vi "Get All VI Data.vi"(8 "error in (no error)":errorcluster, 11 "Path":path) -> (0 "error out":errorcluster, 2 "Displayed Indices":i32[](array[numeric]), 3 "VI Data":T1[](array[typedef]))   [LabVIEW 2023, in "VI Properties Editor.lvlib"]
doc: "Gets all VI data from the source of VIs located at <B>Path</B>."
uses:
  VI Properties Editor.lvlib
  CTLs/VI Data.ctl
  CTLs/VI Properties.ctl
  <vilib>/picture/picture.llb/imagedata.ctl
  CTLs/Control Properties.ctl
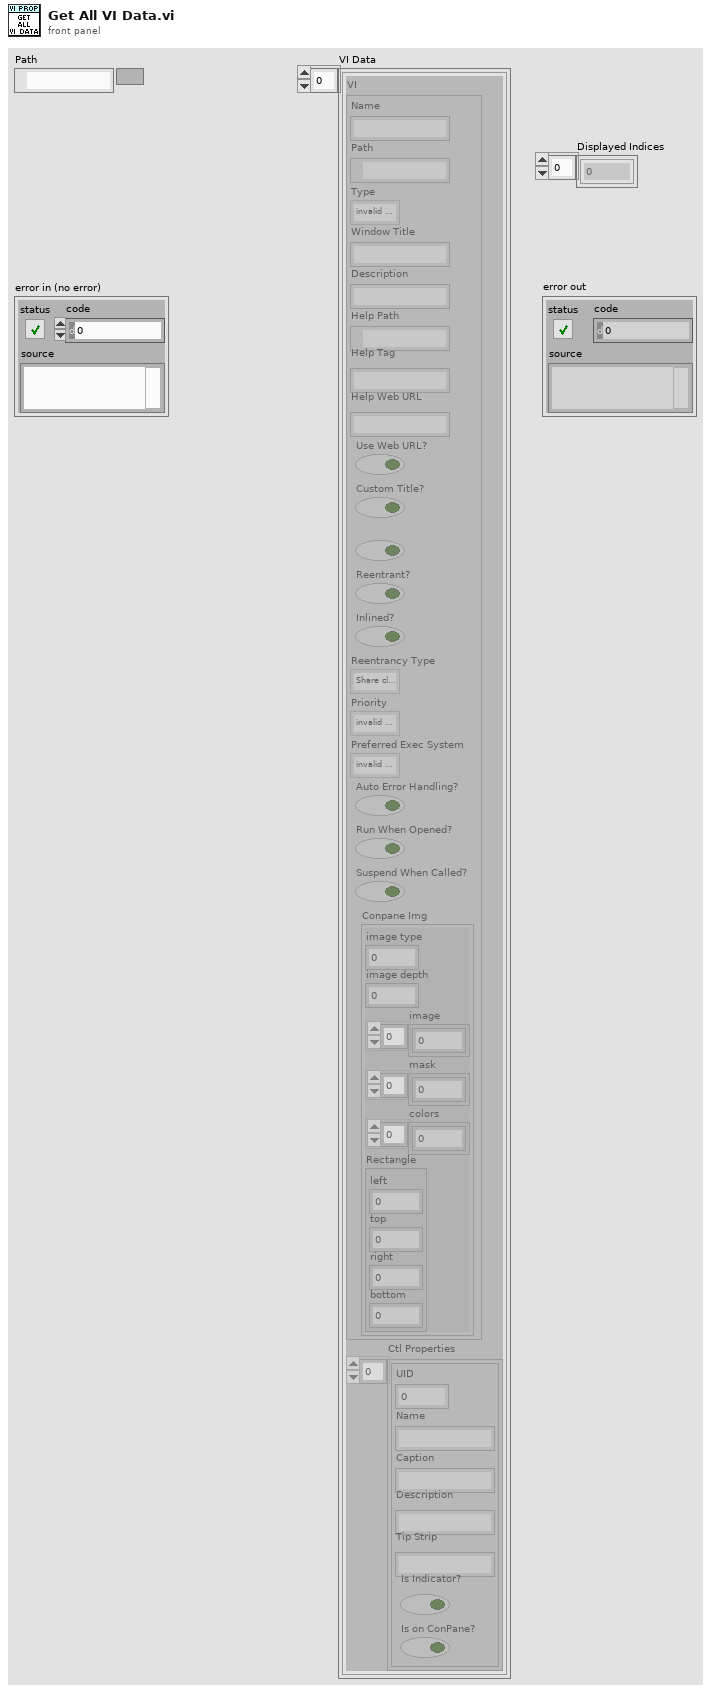
[diagram p1: front panel]
types:
  T1 = typedef "VI Properties Editor.lvlib/VI Data.ctl" = cluster{"VI":T2, "Ctl Properties":T4[]}
  T2 = typedef "VI Properties Editor.lvlib/VI Properties.ctl" = cluster{"Name":string, "Path":path, "Type":enum32{"invalid VI type", "Standard VI", "Control VI", "Global VI", "Polymorphic VI", "Configuration VI", "SubSystem", "Facade VI", "Method VI", "Statechart Diagram VI"}, "Window Title":string, "Description":string, "Help Path":path, "Help Tag":string, "Help Web URL":string, "Use Web URL?":bool, "Custom Title?":bool, "Allow Debugging?":bool, "Reentrant?":bool, "Inlined?":bool, "Reentrancy Type":enum16{"Share clones between instances", "Preallocate clone for each instance"}, "Priority":enum32{"invalid priority", "background priority", "normal priority", "above normal priority", "high priority", "time critical priority", "subroutine"}, "Preferred Exec System":enum32{"invalid execution system", "user interface", "standard", "instrument i/o", "data acquisition", "other 1", "other 2", "same as caller"}, "Auto Error Handling?":bool, "Run When Opened?":bool, "Suspend When Called?":bool, "Conpane Img":T3}
  T3 = typedef "imagedata.ctl" = cluster{"image type":i32, "image depth":i32, "image":u8[], "mask":u8[], "colors":u32[], "Rectangle":cluster{"left":i16, "top":i16, "right":i16, "bottom":i16}}
  T4 = typedef "VI Properties Editor.lvlib/Control Properties.ctl" = cluster{"UID":i32, "Name":string, "Caption":string, "Description":string, "Tip Strip":string, "Is Indicator?":bool, "Is on ConPane?":bool}
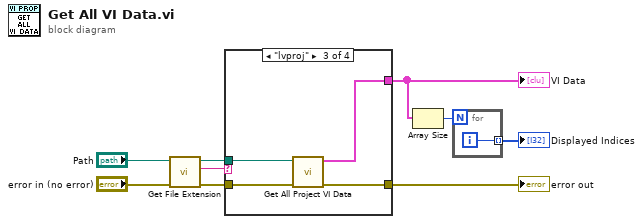
[diagram p0: block diagram]
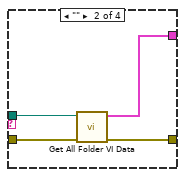
[diagram p3: hidden frame]
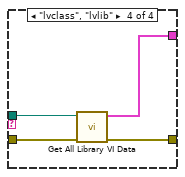
[diagram p4: hidden frame]
diagram:
  n1 = call <vilib>:"Get File Extension.vi"("error in (no error)"="error in (no error)", "file"="Path") -> ("error out"=w5:errorcluster, "lowercase file extension"=w7:string, "dup file"=w6:path)  [unwired: 5 in, 2 out]
  n2 = case shown="\"lvproj\"" w7 {
    tunnel: w6 -> [_ w13 w17 w21]
    tunnel: w5 -> [w10 w14 w18 w22]
    tunnel: [w10 w12 w16 w20] -> w4
    tunnel: [_ w11 w15 w19] -> w3
    frame Default {
    }
    frame "" {
      n3 = call "Get All Folder VI Data.vi"("error in (no error)"=w14, "Path"=w13) -> ("error out"=w12:errorcluster, "VI Data"=w11:T1[])  [unwired: 8 in]
    }
    frame "lvproj" {
      n4 = call "Get All Project VI Data.vi"("error in (no error)"=w18, "Path"=w17) -> ("error out"=w16:errorcluster, "VI Data"=w15:T1[])  [unwired: 8 in]
    }
    frame "lvclass", "lvlib" {
      n5 = call "Get All Library VI Data.vi"("error in (no error)"=w22, "Path"=w21) -> ("error out"=w20:errorcluster, "VI Data"=w19:T1[])  [unwired: 8 in]
    }
  }
  "error out" <- w4
  "VI Data" <- w3
  n6 = Array Size(array=w3) -> (size(s)=w2:i32)
  n7 = for {
    N: w2 -> [_]
    tunnel: [w23] -> w1 mode=indexing
    i -> [w23]
  }
  "Displayed Indices" <- w1
